vi "subValidateBaseContruction.vi"(9 "Parameters":T1, 11 "CLabVIEWItem in":refnum<class "CLabVIEWItem.lvclass">) -> (1 "Actual":T1, 3 "Pass?":bool)   [LabVIEW 2020, in "Tests.LabVIEWItem.lvlib"]
uses:
  Tests.LabVIEWItem.lvlib
  CLabVIEWItem/CLabVIEWItem.lvclass
  Validate_BaseConstruction.ctl
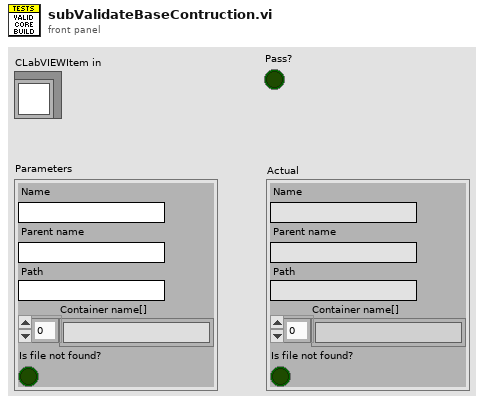
[diagram p1: front panel]
types:
  T1 = typedef "Tests.LabVIEWItem.lvlib/Validate_BaseConstruction.ctl" = cluster{"Name":string, "Parent name":string, "Path":string, "Container name[]":string[], "Is file not found?":bool}
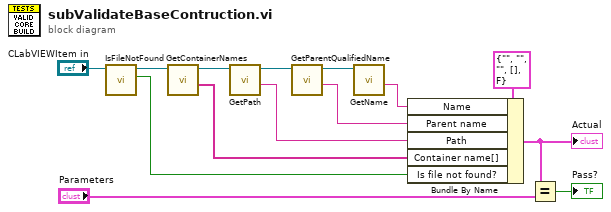
[diagram p0: block diagram]
diagram:
  n1 = call-dynamic "IsFileNotFound.vi"("CLabVIEWItem in"="CLabVIEWItem in") -> ("Is file not found?"=w9:bool, "CLabVIEWItem out"=w4:refnum<class "CLabVIEWItem.lvclass">)  [unwired: 8 in, 1 out]
  n2 = call-dynamic "GetContainerNames.vi"("CLabVIEWItem in"=w4) -> ("Container name[]"=w10:string[], "CLabVIEWItem out"=w3:refnum<class "CLabVIEWItem.lvclass">)  [unwired: 8 in, 1 out]
  n3 = call-dynamic "GetPath.vi"("CLabVIEWItem in"=w3) -> ("Path"=w11:string, "CLabVIEWItem out"=w2:refnum<class "CLabVIEWItem.lvclass">)  [unwired: 8 in, 1 out]
  n4 = call-dynamic "GetParentQualifiedName.vi"("CLabVIEWItem in"=w2) -> ("Name"=w12:string, "CLabVIEWItem out"=w1:refnum<class "CLabVIEWItem.lvclass">)  [unwired: 8 in, 1 out]
  n5 = call-dynamic "GetName.vi"("CLabVIEWItem in"=w1) -> ("Name"=w13:string)  [unwired: 8 in, 2 out]
  n6 = Bundle By Name(cluster=T1 {"Name"="", "Parent name"="", "Path"="", "Container name[]"=[], "Is file not found?"=FALSE} ("Pameters 2"), "Name"=w13, "Parent name"=w12, "Path"=w11, "Container name[]"=w10, "Is file not found?"=w9) -> (w8:T1)
  "Actual" <- w8
  n7 = Equal?(x=w8, y="Parameters") -> (x = y?=→"Pass?":bool)
